vi "Func-엑셀 데이터를 그래프로 출력.vi"() -> ()   [LabVIEW 2015] (continued)
12.421\n3.3\t3.3\t12.426\n3.3\t3.3\t12.427\n3.3\t3.3\t12.425\n3.3\t3.3\t12.423\n3.3\t3.3\t12.423\n3.3\t3.3\t12.418\n3.3\t3.3\t12.419\n3.3\t3.3\t12.42\n3.3\t3.3\t12.421\n3.3\t3.3\t12.42\n3.3\t3.3\t12.418\n3.3\t3.3\t12.415\n3.3\t3.3\t12.414\n3.3\t3.3\t12.41\n3.3\t3.3\t12.41\n3.3\t3.3\t12.409\n3.3\t3.3\t12.411\n3.3\t3.3\t12.414\n3.3\t3.3\t12.414\n3.3\t3.3\t12.415\n3.3\t3.3\t12.412\n3.3\t3.3\t12.415\n3.3\t3.3\t12.413\n3.3\t3.3\t12.408\n3.3\t3.3\t12.406\n3.3\t3.3\t12.404\n3.3\t3.3\t12.408\n3.3\t3.3\t12.406\n3.3\t3.3\t12.408\n3.3\t3.3\t12.411\n3.3\t3.3\t12.412\n3.3\t3.3\t12.413\n3.3\t3.3\t12.413\n3.3\t3.3\t12.412\n3.3\t3.3\t12.41\n3.3\t3.3\t12.407\n3.3\t3.3\t12.409\n3.3\t3.3\t12.407\n3.3\t3.3\t12.401\n3.3\t3.3\t12.402\n3.3\t3.3\t12.405\n3.3\t3.3\t12.406\n3.3\t3.3\t12.405\n3.3\t3.3\t12.407\n3.3\t3.3\t12.41\n3.3\t3.3\t12.408\n3.3\t3.3\t12.407\n3.3\t3.3\t12.407\n3.3\t3.3\t12.405\n3.3\t3.3\t12.404\n3.3\t3.3\t12.402\n3.3\t3.3\t12.402\n3.3\t3.3\t12.398\n3.3\t3.3\t12.395\n3.3\t3.3\t12.396\n3.3\t3.3\t12.395\n3.3\t3.3\t12.395\n3.3\t3.3\t12.393\n3.3\t3.3\t12.396\n3.3\t3.3\t12.399\n3.3\t3.3\t12.4\n3.3\t3.3\t12.4\n3.3\t3.3\t12.398\n3.3\t3.3\t12.398\n3.3\t3.3\t12.396\n3.3\t3.3\t12.398\n3.3\t3.3\t12.396\n3.3\t3.3\t12.398\n3.3\t3.3\t12.396\n3.3\t3.3\t12.396\n3.3\t3.3\t12.393\n3.3\t3.3\t12.391\n3.3\t3.3\t12.391\n3.3\t3.3\t12.389\n3.3\t3.3\t12.389\n3.3\t3.3\t12.391\n3.3\t3.3\t12.395\n3.3\t3.3\t12.394\n3.3\t3.3\t12.391\n3.3\t3.3\t12.39\n3.3\t3.3\t12.391\n3.3\t3.3\t12.39\n3.3\t3.3\t12.384\n3.3\t3.3\t12.384\n3.3\t3.3\t12.386\n3.3\t3.3\t12.382\n3.3\t3.3\t12.385\n3.3\t3.3\t12.384\n3.3\t3.3\t12.387\n3.3\t3.3\t12.39\n3.3\t3.3\t12.39\n3.3\t3.3\t12.393\n3.3\t3.3\t12.387\n3.3\t3.3\t12.385\n3.3\t3.3\t12.384\n3.3\t3.3\t12.379\n3.3\t3.3\t12.376\n3.3\t3.3\t12.376\n3.3\t3.3\t12.379\n3.3\t3.3\t12.377\n3.3\t3.3\t12.376\n3.3\t3.3\t12.379\n3.3\t3.3\t12.383\n3.3\t3.3\t12.386\n3.3\t3.3\t12.387\n3.3\t3.3\t12.391\n3.3\t3.3\t12.387\n3.3\t3.3\t12.388\n3.3\t3.3\t12.389\n3.3\t3.3\t12.385\n3.3\t3.3\t12.382\n3.3\t3.3\t12.382\n3.3\t3.3\t12.384\n3.3\t3.3\t12.381\n3.3\t3.3\t12.381\n3.3\t3.3\t12.38\n3.3\t3.3\t12.385\n3.3\t3.3\t12.38\n3.3\t3.3\t12.379\n3.3\t3.3\t12.379\n3.3\t3.3\t12.377\n3.3\t3.3\t12.377\n3.3\t3.3\t12.373\n3.3\t3.3\t12.374\n3.3\t3.3\t12.373\n3.3\t3.3\t12.373\n3.3\t3.3\t12.371\n3.3\t3.3\t12.366\n3.3\t3.3\t12.365\n3.3\t3.3\t12.366\n3.3\t3.3\t12.364\n3.3\t3.3\t12.365\n3.3\t3.3\t12.364\n3.3\t3.3\t12.371\n3.3\t3.3\t12.372\n3.3\t3.3\t12.375\n3.3\t3.3\t12.375\n3.3\t3.3\t12.376\n3.3\t3.3\t12.378\n3.3\t3.3\t12.376\n3.3\t3.3\t12.379\n3.3\t3.3\t12.375\n3.3\t3.3\t12.375\n3.3\t3.3\t12.372\n3.3\t3.3\t12.372\n3.3\t3.3\t12.371\n3.3\t3.3\t12.369\n3.3\t3.3\t12.37\n3.3\t3.3\t12.368\n3.3\t3.3\t12.371\n3.3\t3.3\t12.37\n3.3\t3.3\t12.365\n3.3\t3.3\t12.364\n3.3\t3.3\t12.365\n3.3\t3.3\t12.364\n3.3\t3.3\t12.361\n3.3\t3.3\t12.359\n3.3\t3.3\t12.364\n3.3\t3.3\t12.365\n3.3\t3.3\t12.365\n3.3\t3.3\t12.362\n3.3\t3.3\t12.361\n3.3\t3.3\t12.365\n3.3\t3.3\t12.364\n3.3\t3.3\t12.361\n3.3\t3.3\t12.361\n3.3\t3.3\t12.367\n3.3\t3.3\t12.37\n3.3\t3.3\t12.368\n3.3\t3.3\t12.369\n3.3\t3.3\t12.37\n3.3\t3.3\t12.367\n3.217\t3.24\t12.192\n3.133\t3.17\t12.187\n3.05\t3.3\t12.191\n2.967\t3.27\t12.191\n2.883\t3.19\t12.188\n2.8\t3.09\t12.182\n2.717\t2.97\t12.183\n2.633\t2.84\t12.189\n2.55\t2.69\t12.18\n2.467\t2.53\t12.185\n2.383\t2.36\t12.183\n2.3\t2.2\t12.179\n2.217\t2.02\t12.179\n2.133\t1.83\t12.175\n2.05\t1.64\t12.17\n1.967\t1.45\t12.171\n1.883\t1.27\t12.168\n1.8\t1.1\t12.165\n1.717\t0.94\t12.155\n1.633\t0.79\t12.159\n1.55\t0.62\t12.146\n1.467\t0.47\t12.139\n1.383\t0.33\t12.134\n1.3\t0.19\t12.124\n1.217\t0.06\t12.113\n1.133\t-0.07\t12.098\n1.05\t-0.19\t12.087\n0.967\t-0.31\t12.078\n0.883\t-0.4\t12.065\n0.8\t-0.49\t12.048\n0.717\t-0.59\t12.022\n0.633\t-0.67\t12.023\n0.55\t-0.78\t12.001\n0.467\t-0.86\t11.98\n0.383\t-0.93\t11.958\n0.3\t-1\t11.937\n0.217\t-1.08\t11.92\n0.133\t-1.16\t11.897\n0.05\t-1.24\t11.874\n-0.033\t-1.3\t11.85\n-0.117\t-1.37\t11.824\n-0.2\t-1.43\t11.798\n-0.283\t-1.52\t11.771\n-0.367\t-1.58\t11.745\n-0.45\t-1.64\t11.715\n-0.533\t-1.72\t11.689\n-0.617\t-1.8\t11.651\n-0.7\t-1.87\t11.626\n-0.783\t-1.95\t11.608\n-0.867\t-2.02\t11.566\n-0.95\t-2.09\t11.538\n-1.033\t-2.15\t11.498\n-1.117\t-2.23\t11.467\n-1.2\t-2.3\t11.441\n-1.283\t-2.39\t11.408\n-1.367\t-2.46\t11.363\n-1.45\t-2.54\t11.333\n-1.533\t-2.62\t11.294\n-1.617\t-2.7\t11.247\n-1.7\t-2.77\t11.214\n-1.783\t-2.84\t11.185\n-1.867\t-2.91\t11.153\n-1.95\t-2.97\t11.105\n-2.033\t-3.05\t11.065\n-2.117\t-3.13\t11.023\n-2.2\t-3.2\t10.986\n-2.283\t-3.27\t10.942\n-2.367\t-3.34\t10.896\n-2.45\t-3.43\t10.852\n-2.533\t-3.52\t10.814\n-2.617\t-3.61\t10.779\n-2.7\t-3.7\t10.737\n-2.783\t-3.79\t10.686\n-2.867\t-3.87\t10.648\n-2.95\t-3.95\t10.597\n-3.033\t-4.04\t10.554\n-3.117\t-4.11\t10.511\n-3.2\t-4.19\t10.461\n-3.283\t-4.28\t10.421\n-3.367\t-4.36\t10.374\n-3.45\t-4.45\t10.324\n-3.533\t-4.53\t10.277\n-3.617\t-4.61\t10.222\n-3.7\t-4.69\t10.18\n-3.783\t-4.77\t10.118\n-3.867\t-4.86\t10.08\n-3.95\t-4.94\t10.032\n-4.033\t-5.02\t9.984\n-4.117\t-5.1\t9.936\n-4.2\t-5.17\t9.882\n-4.283\t-5.24\t9.831\n-4.367\t-5.31\t9.779\n-4.45\t-5.38\t9.728\n-4.533\t-5.46\t9.677\n-4.617\t-5.54\t9.633\n-4.7\t-5.63\t9.577\n-4.783\t-5.71\t9.515\n-4.867\t-5.78\t9.462\n-4.95\t-5.85\t9.406\n-5.033\t-5.94\t9.355\n-5.117\t-6.01\t9.297\n-5.2\t-6.1\t9.244\n-5.283\t-6.18\t9.196\n-5.367\t-6.26\t9.14\n-5.45\t-6.34\t9.087\n-5.533\t-6.43\t9.022\n-5.617\t-6.51\t8.968\n-5.7\t-6.61\t8.91\n-5.783\t-6.69\t8.852\n-5.867\t-6.77\t8.798\n-5.95\t-6.84\t8.734\n-6.033\t-6.91\t8.679\n-6.117\t-7\t8.621\n-6.2\t-7.07\t8.569\n-6.283\t-7.15\t8.51\n-6.367\t-7.23\t8.45\n-6.45\t-7.31\t8.386\n-6.533\t-7.39\t8.33\n-6.617\t-7.47\t8.273\n-6.7\t-7.55\t8.211\n-6.783\t-7.64\t8.148\n-6.867\t-7.71\t8.092\n-6.95\t-7.78\t8.034\n-7.033\t-7.85\t7.975\n-7.117\t-7.94\t7.92\n-7.2\t-8.03\t7.855\n-7.283\t-8.11\t7.796\n-7.367\t-8.2\t7.736\n-7.45\t-8.27\t7.664\n-7.533\t-8.34\t7.6\n-7.617\t-8.41\t7.547\n-7.7\t-8.49\t7.482\n-7.783\t-8.58\t7.42\n-7.867\t-8.65\t7.364\n-7.95\t-8.71\t7.293\n-8.033\t-8.79\t7.231\n-8.117\t-8.87\t7.175\n-8.2\t-8.96\t7.106\n-8.283\t-9.04\t7.051\n-8.367\t-9.13\t6.983\n-8.45\t-9.21\t6.926\n-8.533\t-9.28\t6.858\n-8.617\t-9.38\t6.793\n-8.7\t-9.47\t6.727\n-8.783\t-9.56\t6.664\n-8.867\t-9.63\t6.597\n-8.95\t-9.7\t6.531\n-9.033\t-9.78\t6.471\n-9.117\t-9.85\t6.404\n-9.2\t-9.93\t6.333\n-9.283\t-10.01\t6.27\n-9.367\t-10.09\t6.204\n-9.45\t-10.16\t6.137\n-9.533\t-10.23\t6.075\n-9.617\t-10.29\t5.998\n-9.7\t-10.37\t5.934\n-9.783\t-10.45\t5.87\n-9.867\t-10.51\t5.819\n-9.95\t-10.59\t5.74\n-10.033\t-10.66\t5.668\n-10.117\t-10.77\t5.608\n-10.2\t-10.85\t5.535\n-10.283\t-10.92\t5.477\n-10.367\t-11.01\t5.404\n-10.45\t-11.08\t5.328\n-10.533\t-11.16\t5.268\n-10.617\t-11.25\t5.187\n-10.7\t-11.34\t5.126\n-10.783\t-11.44\t5.054\n-10.867\t-11.51\t4.991\n-10.95\t-11.59\t4.914\n-11.033\t-11.67\t4.848\n-11.117\t-11.76\t4.791\n-11.2\t-11.83\t4.719\n-11.283\t-11.9\t4.646\n-11.367\t-11.97\t4.574\n-11.45\t-12.05\t4.513\n-11.533\t-12.13\t4.448\n-11.617\t-12.2\t4.376\n-11.7\t-12.29\t4.3\n-11.783\t-12.38\t4.225\n-11.867\t-12.45\t4.166\n-11.95\t-12.53\t4.096\n-12.033\t-12.6\t4.03\n-12.117\t-12.68\t3.954\n-12.2\t-12.77\t3.891\n-12.283\t-12.86\t3.822\n-12.367\t-12.94\t3.746\n-12.45\t-13.01\t3.677\n-12.533\t-13.09\t3.613\n-12.617\t-13.16\t3.542\n-12.7\t-13.25\t3.473\n-12.783\t-13.34\t3.404\n-12.867\t-13.42\t3.329\n-12.95\t-13.48\t3.254\n-13.033\t-13.56\t3.193\n-13.117\t-13.64\t3.113\n-13.2\t-13.71\t3.046\n-13.283\t-13.79\t2.978\n-13.367\t-13.87\t2.907\n-13.45\t-13.95\t2.842\n-13.533\t-14.03\t2.765\n-13.617\t-14.11\t2.7\n-13.7\t-14.18\t2.624\n-13.783\t-14.27\t2.555\n-13.867\t-14.34\t2.485\n-13.95\t-14.41\t2.421\n-14.033\t-14.5\t2.347\n-14.117\t-14.57\t2.266\n-14.2\t-14.64\t2.201\n-14.283\t-14.72\t2.132\n-14.367\t-14.8\t2.056\n-14.45\t-14.89\t1.991\n-14.533\t-14.97\t1.922\n-14.617\t-15.05\t1.845\n-14.7\t-15.14\t1.77\n-14.783\t-15.23\t1.703\n-14.867\t-15.31\t1.634\n-14.95\t-15.4\t1.557\n-15.033\t-15.48\t1.484\n-15.117\t-15.57\t1.413\n-15.2\t-15.65\t1.337\n-15.283\t-15.74\t1.263\n-15.367\t-15.82\t1.198\n-15.45\t-15.89\t1.124\n-15.533\t-15.97\t1.05\n-15.617\t-16.04\t0.985\n-15.7\t-16.12\t0.899\n-15.783\t-16.21\t0.833\n-15.867\t-16.28\t0.753\n-15.95\t-16.37\t0.682\n-16.033\t-16.44\t0.606\n-16.117\t-16.52\t0.537\n-16.2\t-16.6\t0.459\n-16.283\t-16.7\t0.39\n-16.367\t-16.78\t0.321\n-16.45\t-16.86\t0.246\n-16.533\t-16.95\t0.177\n-16.617\t-17.03\t0.086\n-16.7\t-17.11\t0.024\n-16.783\t-17.18\t-0.057\n-16.867\t-17.26\t-0.131\n-16.95\t-17.32\t-0.202\n-17.033\t-17.4\t-0.277\n-17.117\t-17.47\t-0.355\n-17.2\t-17.55\t-0.428\n-17.283\t-17.63\t-0.502\n-17.367\t-17.72\t-0.575\n-17.45\t-17.8\t-0.648\n-17.533\t-17.88\t-0.723\n-17.617\t-17.96\t-0.79\n-17.7\t-18.04\t-0.882\n-17.783\t-18.12\t-0.951\n-17.867\t-18.2\t-1.024\n-17.95\t-18.28\t-1.102\n-18.033\t-18.35\t-1.17\n-18.117\t-18.42\t-1.246\n-18.2\t-18.49\t-1.317\n-18.283\t-18.58\t-1.407\n-18.367\t-18.66\t-1.468\n-18.3\t-18.73\t-1.546\n-18.3\t-18.74\t-1.555\n-18.3\t-18.75\t-1.559\n-18.3\t-18.75\t-1.568\n-18.3\t-18.76\t-1.578\n-18.3\t-18.77\t-1.583\n-18.3\t-18.78\t-1.591\n-18.3\t-18.79\t-1.598\n-18.3\t-18.8\t-1.603\n-18.3\t-18.81\t-1.607\n-18.3\t-18.82\t-1.611\n-18.3\t-18.82\t-1.618\n-18.3\t-18.83\t-1.622\n-18.3\t-18.84\t-1.633\n-18.3\t-18.85\t-1.641\n-18.3\t-18.86\t-1.648\n-18.3\t-18.87\t-1.659\n-18.3\t-18.87\t-1.662\n-18.3\t-18.88\t-1.671\n-18.3\t-18.89\t-1.678\n-18.3\t-18.9\t-1.686\n-18.3\t-18.9\t-1.695\n-18.3\t-18.91\t-1.704\n-18.3\t-18.92\t-1.715\n-18.3\t-18.93\t-1.723\n-18.3\t-18.94\t-1.735\n-18.3\t-18.95\t-1.739\n-18.3\t-18.95\t-1.746\n-18.3\t-18.96\t-1.755\n-18.3\t-18.97\t-1.761\n-18.3\t-18.98\t-1.766\n-18.3\t-18.99\t-1.773\n-18.3\t-18.99\t-1.783\n-18.3\t-19\t-1.788\n-18.3\t-19.01\t-1.801\n-18.3\t-19.02\t-1.809\n-18.3\t-19.03\t-1.82\n-18.3\t-19.03\t-1.829\n-18.3\t-19.04\t-1.835\n-18.3\t-19.05\t-1.845\n-18.3\t-19.06\t-1.848\n-18.3\t-19.06\t-1.853\n-18.3\t-19.06\t-1.86\n-18.3\t-19.07\t-1.871\n-18.3\t-19.08\t-1.877\n-18.3\t-19.08\t-1.887\n-18.3\t-19.09\t-1.893\n-18.3\t-19.1\t-1.904\n-18.3\t-19.1\t-1.911\n-18.3\t-19.11\t-1.917\n-18.3\t-19.11\t-1.925\n-18.3\t-19.12\t-1.932\n-18.3\t-19.13\t-1.939\n-18.3\t-19.14\t-1.947\n-18.3\t-19.14\t-1.954\n-18.3\t-19.14\t-1.959\n-18.3\t-19.14\t-1.962\n-18.3\t-19.15\t-1.976\n-18.3\t-19.16\t-1.984\n-18.3\t-19.16\t-1.987\n-18.3\t-19.17\t-1.999\n-18.3\t-19.17\t-2.007\n-18.3\t-19.18\t-2.016\n-18.3\t-19.18\t-2.024\n-18.3\t-19.18\t-2.029\n-18.3\t-19.19\t-2.039\n-18.3\t-19.19\t-2.046\n-18.3\t-19.19\t-2.055\n-18.3\t-19.19\t-2.063\n-18.3\t-19.2\t-2.071\n-18.3\t-19.21\t-2.076\n-18.3\t-19.21\t-2.081\n-18.3\t-19.22\t-2.091\n-18.3\t-19.22\t-2.096\n-18.3\t-19.22\t-2.102\n-18.3\t-19.22\t-2.11\n-18.3\t-19.22\t-2.122\n-18.3\t-19.23\t-2.128\n-18.3\t-19.23\t-2.136\n-18.3\t-19.23\t-2.143\n-18.3\t-19.24\t-2.152\n-18.3\t-19.24\t-2.158\n-18.3\t-19.25\t-2.166\n-18.3\t-19.25\t-2.175\n-18.3\t-19.25\t-2.18\n-18.3\t-19.26\t-2.188\n-18.3\t-19.26\t-2.192\n-18.3\t-19.26\t-2.203\n-18.3\t-19.26\t-2.209\n-18.3\t-19.26\t-2.215\n-18.3\t-19.27\t-2.226\n-18.3\t-19.27\t-2.236\n-18.3\t-19.27\t-2.245\n-18.3\t-19.27\t-2.25\n-18.3\t-19.27\t-2.261\n-18.3\t-19.28\t-2.266\n-18.3\t-19.28\t-2.272\n-18.3\t-19.28\t-2.283\n-18.3\t-19.28\t-2.291\n-18.3\t-19.28\t-2.298\n-18.3\t-19.28\t-2.306\n-18.3\t-19.28\t-2.315\n-18.3\t-19.28\t-2.319\n-18.3\t-19.28\t-2.327\n-18.3\t-19.28\t-2.329\n-18.3\t-19.28\t-2.337\n-18.3\t-19.28\t-2.343\n-18.3\t-19.28\t-2.35\n-18.3\t-19.28\t-2.362\n-18.3\t-19.28\t-2.371\n-18.3\t-19.28\t-2.38\n-18.3\t-19.28\t-2.388\n-18.3\t-19.28\t-2.398\n-18.3\t-19.28\t-2.403\n-18.3\t-19.28\t-2.407\n-18.3\t-19.28\t-2.417\n-18.3\t-19.28\t-2.425\n-18.3\t-19.29\t-2.429\n-18.3\t-19.29\t-2.439\n-18.3\t-19.29\t-2.446\n-18.3\t-19.29\t-2.45\n-18.3\t-19.29\t-2.458\n-18.3\t-19.29\t-2.461\n-18.3\t-19.29\t-2.469\n-18.3\t-19.29\t-2.476\n-18.3\t-19.29\t-2.483\n-18.3\t-19.29\t-2.489\n-18.3\t-19.29\t-2.496\n-18.3\t-19.29\t-2.503\n-18.3\t-19.29\t-2.509\n-18.3\t-19.29\t-2.519\n-18.3\t-19.29\t-2.525\n-18.3\t-19.29\t-2.535\n-18.3\t-19.29\t-2.547\n-18.3\t-19.28\t-2.554\n-18.3\t-19.29\t-2.564\n-18.3\t-19.28\t-2.572\n-18.3\t-19.28\t-2.579\n-18.3\t-19.28\t-2.583\n-18.3\t-19.28\t-2.593\n-18.3\t-19.27\t-2.605\n-18.3\t-19.28\t-2.614\n-18.3\t-19.28\t-2.621\n-18.3\t-19.28\t-2.629\n-18.3\t-19.28\t-2.64\n-18.3\t-19.28\t-2.648\n-18.3\t-19.28\t-2.652\n-18.3\t-19.27\t-2.659\n-18.3\t-19.27\t-2.667\n-18.3\t-19.27\t-2.673\n-18.3\t-19.28\t-2.677\n-18.3\t-19.28\t-2.682\n-18.3\t-19.28\t-2.687\n-18.3\t-19.27\t-2.696\n-18.3\t-19.27\t-2.701\n-18.3\t-19.27\t-2.708\n-18.3\t-19.27\t-2.719\n-18.3\t-19.26\t-2.724\n-18.3\t-19.26\t-2.734\n-18.3\t-19.26\t-2.743\n-18.3\t-19.26\t-2.751\n-18.3\t-19.27\t-2.754\n-18.3\t-19.26\t-2.765\n-18.3\t-19.26\t-2.774\n-18.3\t-19.26\t-2.78\n-18.3\t-19.26\t-2.789\n-18.3\t-19.26\t-2.794\n-18.3\t-19.26\t-2.804\n-18.3\t-19.26\t-2.814\n-18.3\t-19.26\t-2.821\n-18.3\t-19.26\t-2.829\n-18.3\t-19.25\t-2.84\n-18.3\t-19.25\t-2.845\n-18.3\t-19.25\t-2.852\n-18.3\t-19.25\t-2.86\n-18.3\t-19.25\t-2.867\n-18.3\t-19.25\t-2.871\n-18.3\t-19.25\t-2.879\n-18.3\t-19.24\t-2.884\n-18.3\t-19.24\t-2.891\n-18.3\t-19.24\t-2.897\n-18.3\t-19.23\t-2.901\n-18.3\t-19.23\t-2.908\n-18.3\t-19.24\t-2.916\n-18.3\t-19.24\t-2.925\n-18.3\t-19.24\t-2.93\n-18.3\t-19.24\t-2.942\n-18.3\t-19.23\t-2.95\n-18.3\t-19.23\t-2.959\n-18.3\t-19.23\t-2.97\n-18.3\t-19.23\t-2.975\n-18.3\t-19.23\t-2.98\n-18.3\t-19.22\t-2.989\n-18.3\t-19.22\t-2.996\n-18.3\t-19.22\t-3.002\n-18.3\t-19.22\t-3.013\n-18.3\t-19.22\t-3.022\n-18.3\t-19.22\t-3.031\n-18.3\t-19.22\t-3.037\n-18.3\t-19.21\t-3.043\n-18.3\t-19.21\t-3.049\n-18.3\t-19.21\t-3.052\n-18.3\t-19.21\t-3.055\n-18.3\t-19.21\t-3.064\n-18.3\t-19.21\t-3.074\n-18.3\t-19.21\t-3.081\n-18.3\t-19.2\t-3.088\n-18.3\t-19.2\t-3.096\n-18.3\t-19.2\t-3.105\n-18.3\t-19.2\t-3.112\n-18.3\t-19.19\t-3.115\n-18.3\t-19.19\t-3.122\n-18.3\t-19.19\t-3.132\n-18.3\t-19.19\t-3.139\n-18.3\t-19.19\t-3.145\n-18.3\t-19.19\t-3.154\n-18.3\t-19.19\t-3.165\n-18.3\t-19.19\t-3.171\n-18.3\t-19.19\t-3.177\n-18.3\t-19.18\t-3.184\n-18.3\t-19.18\t-3.189\n-18.3\t-19.18\t-3.196\n-18.3\t-19.17\t-3.203\n-18.3\t-19.17\t-3.208\n-18.3\t-19.17\t-3.214\n-18.3\t-19.17\t-3.222\n-18.3\t-19.16\t-3.229\n-18.3\t-19.16\t-3.241\n-18.3\t-19.15\t-3.251\n-18.3\t-19.15\t-3.26\n-18.3\t-19.14\t-3.267\n-18.3\t-19.14\t-3.277\n-18.3\t-19.14\t-3.282\n-18.3\t-19.14\t-3.286\n-18.3\t-19.14\t-3.294\n-18.3\t-19.14\t-3.299\n-18.3\t-19.14\t-3.308\n-18.3\t-19.13\t-3.32\n-18.3\t-19.13\t-3.329\n-18.3\t-19.13\t-3.338\n-18.3\t-19.12\t-3.343\n-18.3\t-19.12\t-3.35\n-18.3\t-19.11\t-3.356\n-18.3\t-19.11\t-3.359\n-18.3\t-19.11\t-3.365\n-18.3\t-19.1\t-3.372\n-18.3\t-19.1\t-3.378\n-18.3\t-19.09\t-3.386\n-18.3\t-19.09\t-3.395\n-18.3\t-19.08\t-3.399\n-18.3\t-19.08\t-3.407\n-18.3\t-19.07\t-3.416\n-18.3\t-19.07\t-3.421\n-18.3\t-19.06\t-3.425\n-18.3\t-19.06\t-3.436\n-18.3\t-19.06\t-3.448\n-18.3\t-19.06\t-3.454\n-18.3\t-19.05\t-3.464\n-18.3\t-19.05\t-3.474\n-18.3\t-19.04\t-3.483\n-18.3\t-19.04\t-3.49\n-18.3\t-19.03\t-3.492\n-18.3\t-19.03\t-3.496\n-18.3\t-19.03\t-3.504\n-18.3\t-19.02\t-3.507\n-18.3\t-19.02\t-3.512\n-18.3\t-19.01\t-3.519\n-18.3\t-19.01\t-3.525\n-18.3\t-19\t-3.534\n-18.3\t-19\t-3.543\n-18.3\t-18.99\t-3.548\n-18.3\t-18.99\t-3.553\n-18.3\t-18.99\t-3.56\n-18.3\t-18.99\t-3.57\n-18.3\t-18.98\t-3.574\n-18.3\t-18.98\t-3.58\n-18.3\t-18.97\t-3.588\n-18.3\t-18.97\t-3.596\n-18.3\t-18.96\t-3.606\n-18.3\t-18.96\t-3.611\n-18.3\t-18.96\t-3.619\n-18.3\t-18.96\t-3.629\n-18.3\t-18.95\t-3.636\n-18.3\t-18.95\t-3.644\n-18.3\t-18.94\t-3.654\n-18.3\t-18.94\t-3.659\n-18.3\t-18.93\t-3.668\n-18.3\t-18.92\t-3.675\n-18.3\t-18.92\t-3.681\n-18.3\t-18.92\t-3.688\n-18.3\t-18.91\t-3.698\n-18.3\t-18.91\t-3.707\n-18.3\t-18.91\t-3.714\n-18.3\t-18.9\t-3.721\n-18.3\t-18.9\t-3.728\n-18.3\t-18.9\t-3.732\n-18.3\t-18.9\t-3.737\n-18.3\t-18.89\t-3.741\n-18.3\t-18.89\t-3.749\n-18.3\t-18.89\t-3.756\n-18.3\t-18.89\t-3.759\n-18.3\t-18.89\t-3.77\n-18.3\t-18.9\t-3.777\n-18.3\t-18.89\t-3.781\n-18.3\t-18.89\t-3.792\n-18.3\t-18.88\t-3.797\n-18.3\t-18.88\t-3.805\n-18.3\t-18.87\t-3.813\n-18.3\t-18.87\t-3.82\n-18.3\t-18.87\t-3.827\n-18.3\t-18.86\t-3.83\n-18.3\t-18.87\t-3.835\n-18.3\t-18.86\t-3.841\n-18.3\t-18.86\t-3.849\n-18.3\t-18.86\t-3.851\n-18.3\t-18.85\t-3.859\n-18.3\t-18.85\t-3.866\n-18.3\t-18.84\t-3.871\n-18.3\t-18.84\t-3.878\n-18.3\t-18.84\t-3.889\n-18.3\t-18.83\t-3.896\n-18.3\t-18.83\t-3.9\n-18.3\t-18.83\t-3.913\n-18.3\t-18.83\t-3.922\n-18.3\t-18.83\t-3.929\n-18.3\t-18.82\t-3.932\n-18.3\t-18.82\t-3.941\n-18.3\t-18.82\t-3.949\n-18.3\t-18.82\t-3.954\n-18.3\t-18.82\t-3.958\n-18.3\t-18.81\t-3.959\n-18.3\t-18.81\t-3.97\n-18.3\t-18.81\t-3.978\n-18.3\t-18.8\t-3.984\n-18.3\t-18.8\t-3.996\n-18.3\t-18.8\t-4.005\n-18.3\t-18.79\t-4.014\n-18.3\t-18.79\t-4.021\n-18.3\t-18.79\t-4.021\n-18.3\t-18.78\t-4.027\n-18.3\t-18.78\t-4.035\n-18.3\t-18.78\t-4.041\n-18.3\t-18.77\t-4.046\n-18.3\t-18.77\t-4.052\n-18.3\t-18.76\t-4.059\n-18.3\t-18.76\t-4.067\n-18.3\t-18.75\t-4.073\n-18.3\t-18.75\t-4.082\n-18.3\t-18.75\t-4.086\n-18.3\t-18.75\t-4.095\n-18.3\t-18.75\t-4.104\n-18.3\t-18.75\t-4.108\n-18.3\t-18.75\t-4.118\n-18.3\t-18.75\t-4.121\n-18.3\t-18.74\t-4.13\n-18.3\t-18.74\t-4.137\n-18.3\t-18.73\t-4.142\n-18.3\t-18.73\t-4.146\n-18.3\t-18.72\t-4.151\n-18.3\t-18.72\t-4.156\n-18.3\t-18.72\t-4.156\n-18.3\t-18.71\t-4.162\n-18.3\t-18.71\t-4.169\n-18.3\t-18.71\t-4.179\n-18.3\t-18.71\t-4.187\n-18.3\t-18.7\t-4.196\n-18.3\t-18.7\t-4.207\n-18.3\t-18.7\t-4.22\n-18.3\t-18.69\t-4.222\n-18.3\t-18.69\t-4.225\n-18.3\t-18.68\t-4.234\n-18.3\t-18.68\t-4.238\n-18.3\t-18.68\t-4.244\n-18.3\t-18.67\t-4.248\n-18.3\t-18.67\t-4.256\n-18.3\t-18.67\t-4.261\n-18.3\t-18.67\t-4.266\n-18.3\t-18.67\t-4.272\n-18.3\t-18.66\t-4.274\n-18.3\t-18.66\t-4.279\n-18.3\t-18.65\t-4.282\n-18.3\t-18.65\t-4.288\n-18.3\t-18.64\t-4.297\n-18.3\t-18.64\t-4.3\n-18.3\t-18.63\t-4.311\n-18.3\t-18.63\t-4.322\n-18.3\t-18.63\t-4.328\n-18.3\t-18.62\t-4.336\n-18.3\t-18.62\t-4.343\n-18.3\t-18.62\t-4.35\n-18.3\t-18.61\t-4.357\n-18.3\t-18.61\t-4.364\n-18.3\t-18.6\t-4.376\n-18.3\t-18.6\t-4.38\n-18.3\t-18.6\t-4.386\n-18.3\t-18.6\t-4.391\n-18.3\t-18.59\t-4.396\n-18.3\t-18.59\t-4.402\n-18.3\t-18.59\t-4.404\n-18.3\t-18.59\t-4.409\n-18.3\t-18.59\t-4.416\n-18.3\t-18.59\t-4.423\n-18.3\t-18.58\t-4.424\n-18.3\t-18.58\t-4.434\n-18.3\t-18.57\t-4.44\n-18.3\t-18.57\t-4.445\n-18.3\t-18.57\t-4.45\n-18.3\t-18.57\t-4.455\n-18.3\t-18.56\t-4.464\n-18.3\t-18.56\t-4.47\n-18.3\t-18.56\t-4.475\n-18.3\t-18.56\t-4.479\n-18.3\t-18.56\t-4.489\n-18.3\t-18.56\t-4.495\n-18.3\t-18.55\t-4.5\n-18.3\t-18.55\t-4.509\n-18.3\t-18.55\t-4.515\n-18.3\t-18.54\t-4.521\n-18.3\t-18.54\t-4.532\n-18.3\t-18.54\t-4.536\n-18.3\t-18.54\t-4.54\n-18.3\t-18.53\t-4.545\n-18.3\t-18.53\t-4.552\n-18.3\t-18.53\t-4.556\n-18.3\t-18.52\t-4.562\n-18.3\t-18.52\t-4.568\n-18.3\t-18.51\t-4.574\n-18.3\t-18.51\t-4.582\n-18.3\t-18.51\t-4.586\n-18.3\t-18.51\t-4.595\n-18.3\t-18.51\t-4.6\n-18.3\t-18.51\t-4.603\n-18.3\t-18.5\t-4.609\n-18.3\t-18.5\t-4.613\n-18.3\t-18.49\t-4.618\n-18.3\t-18.49\t-4.623\n-18.3\t-18.49\t-4.63\n-18.3\t-18.49\t-4.636\n-18.3\t-18.49\t-4.643\n-18.3\t-18.49\t-4.652\n-18.3\t-18.49\t-4.66\n-18.3\t-18.48\t-4.664\n-18.3\t-18.48\t-4.672\n-18.3\t-18.47\t-4.677\n-18.3\t-18.47\t-4.682\n-18.3\t-18.46\t-4.687\n-18.3\t-18.46\t-4.691\n-18.3\t-18.46\t-4.702\n-18.3\t-18.45\t-4.708\n-18.3\t-18.45\t-4.715\n-18.3\t-18.45\t-4.721\n-18.3\t-18.45\t-4.728\n-18.3\t-18.45\t-4.731\n-18.3\t-18.44\t-4.736\n-18.3\t-18.44\t-4.741\n-18.3\t-18.44\t-4.747\n-18.3\t-18.44\t-4.751\n-18.3\t-18.43\t-4.76\n-18.3\t-18.43\t-4.766\n-18.3\t-18.43\t-4.772\n-18.3\t-18.43\t-4.776\n-18.3\t-18.43\t-4.779\n-18.3\t-18.43\t-4.782\n-18.3\t-18.43\t-4.786\n-18.3\t-18.43\t-4.791\n-18.3\t-18.43\t-4.794\n-18.3\t-18.43\t-4.802\n-18.3\t-18.43\t-4.806\n-18.3\t-18.43\t-4.816\n-18.3\t-18.43\t-4.825\n-18.3\t-18.43\t-4.829\n-18.3\t-18.43\t-4.839\n-18.3\t-18.43\t-4.842\n-18.3\t-18.42\t-4.846\n-18.3\t-18.41\t-4.846\n-18.3\t-18.4\t-4.85\n-18.3\t-18.39\t-4.855\n-18.3\t-18.38\t-4.857\n-18.3\t-18.37\t-4.866\n-18.3\t-18.36\t-4.875\n-18.3\t-18.35\t-4.883\n-18.3\t-18.34\t-4.891\n-18.3\t-18.33\t-4.898\n-18.3\t-18.32\t-4.905\n-18.3\t-18.31\t-4.914\n-18.3\t-18.33\t-4.917\n-18.3\t-18.32\t-4.924\n-18.3\t-18.32\t
